vi "Write Monitor Data to Host.vi"(11 "Monitor Data Cluster":T1) -> (3 "Overflow?":bool)   [LabVIEW 2016]
uses:
  Typedefs/Monitor Data Cluster.ctl
  <vilib>/rvi/interface/RandomDataEmulation/niFpgaRandomDataHandleErrors.vi
  <vilib>/rvi/DataTransferAndStorage/Container/XNode/niFpgaContainer.xnode
  <vilib>/rvi/interface/RandomDataEmulation/nirviRandomDataFpgaReadWriteTemplate.vi
  Host/Typedefs/IO Buffer Operation.ctl
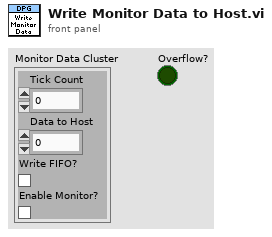
[diagram p1: front panel]
types:
  T1 = typedef "Monitor Data Cluster.ctl" = cluster{"Tick Count":u32, "Data to Host":u64, "Write FIFO?":bool, "Enable Monitor?":bool}
  T2 = typedef "IO Buffer Operation.ctl" = enum16{"Initialize", "Write IO Data_Rd", "Read IO Data_Rd", "Write IO Data_Wr", "Read IO Data_Wr", "Write  IO Data_Dir", "Read  IO Data_Dir", "Write Host to Target FIFO", "Read Host to Target FIFO", "Write Target to Host FIFO", "Read Target to Host FIFO", "Write Monitor Enable?", "Read Monitor Enable?", "Close"}
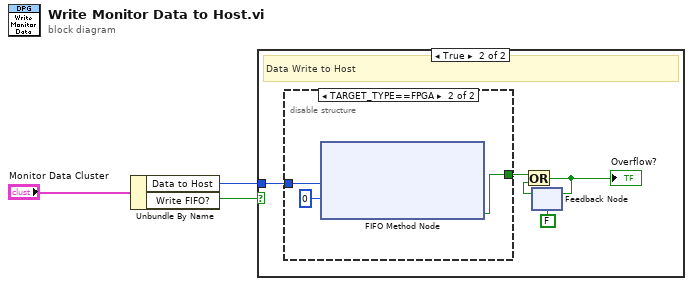
[diagram p0: block diagram]
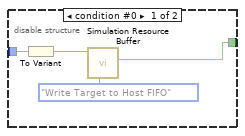
[diagram p3: hidden frame]
diagram:
  n1 = Unbundle By Name("Monitor Data Cluster") -> ("Data to Host"=w2:u64, "Write FIFO?"=w1:bool)
  n2 = case shown="True" w1 {
    tunnel: w2 -> [_ w8]
    frame False {
    }
    frame True {
      # "Data Write to Host"
      n3 = disable-structure shown="TARGET_TYPE==FPGA" {
        disable-tunnel: w8 -> [w11 w15]
        disable-tunnel: [w9 w13] -> w5
        frame condition #0 {
          n4 = To Variant(anything=w11) -> (Variant=w10:variant)
          n5 = call "Simulation Resource Buffer.vi"("IO Buffer Operation"=IO_Buffer_Operation."Write Target to Host FIFO", "Data in"=w10) -> ("Timed Out?"=w9:bool)  [unwired: 7 in, 2 out]
        }
        frame condition #1 (active) {
          n6 = xnode ("FIFO Method Node")("Element"=w15, "Timeout"=0) -> ("Timed Out?"=w13:bool)  [unwired: 1 in, 1 out]
        }
      }
      n7 = feedback #1(FALSE ("Timed Out?")) -> (w6:bool)
      n8 = Or(x=w5, y=w6) -> (x .or. y?=w4:bool)
      "Overflow?" <- w4
      n9 = feedback-in #1(w4) -> ()
    }
  }
